vi "Test Server.vi"() -> ()   [LabVIEW 2013]
uses:
  FPGA/Rate.ctl
  <vilib>/rvi/interface/common/niFpgaWaitOnOcc.vi
  <vilib>/FPGAPlugInAG/sbRIO-9606/niLvFpga_Open_sbRIO-9606.vi
  <vilib>/rvi/interface/common/dynamic/niFpgaDynamicAddResources.vi
  <vilib>/Utility/error.llb/Error Cluster From Error Code.vi
  <vilib>/rvi/errors/niLvFpgaAdjustHostInterfaceError.vi
  <vilib>/FPGAPlugInAG/Dynamic/niLvFpga_Close_Dynamic.vi
  <vilib>/rvi/interface/nirviOpenFPGA/nirviOpenFPGA.xnode
  FPGA Bitfiles/Timothy.lvbitx
  <vilib>/rvi/interface/nirviMethod/nirviMethod.xnode
  <vilib>/rvi/interface/nirviReadWriteControl/nirviReadWriteControl.xnode
  <vilib>/rvi/interface/nirviCloseFPGA/nirviCloseFPGA.xnode
  <vilib>/rvi/errors/niLvFpgaMergeErrorWithErrorCode.vi
  <vilib>/rvi/interface/Simulation/niFpgaSimulationCallBeginRW.vi
  NiFpgaLv.dll
  <vilib>/FPGAPlugInAG/Dynamic/niLvFpga_ReadFifo_Dynamic.vi
  <vilib>/Analysis/NI_AALBase.lvlib
  Reusable/General/Math Utilities.lvlib
  <vilib>/FPGAPlugInAG/Dynamic/niLvFpga_ConfigureFifo_Dynamic.vi
  <vilib>/FPGAPlugInAG/Dynamic/niLvFpga_StartFifo_Dynamic.vi
panel:
  out "Waveform Graph 3":dbl[](graph)
  out "Delay Ticks":u32
  in  "Delay (us)":u16=16
  in  "element":dbl=16.0 format="%#_13g"
  in  "index (row)":i32
  out "Waveform Chart":cluster{i32, i32}(graph)={-1, -1}
  out "max index(es) 2":i32=-1
  out "max index(es)":i32=-1
  in  "right rank":i32=3
  out "Waveform Graph 2":i16[](graph)
  out "Exe Rate (ms)":u32=10121
  in  "Sample Time (us)":u16=100
  out "Sample Time Actual":u32
  in  "Rate":T1=8 items=["2.5 MHz"=8, "5 MHz"=4, "10 MHz"=2, "20MHz"=1]
  out "XY Graph":cluster{dbl[], dbl[]}[](graph)=[{[], []}, {[16.0, 16.0], [0.0, 0.0]}]
  out "dNewData":u64
  out "NumElements":u32
  out "samp/cycle":dbl=nan
  out "dSamps":u64
  out "Samps":u64
  in  "NumSamps":u32=100000
  out "Actual Depth":u32=1000000
  in  "Stop":bool
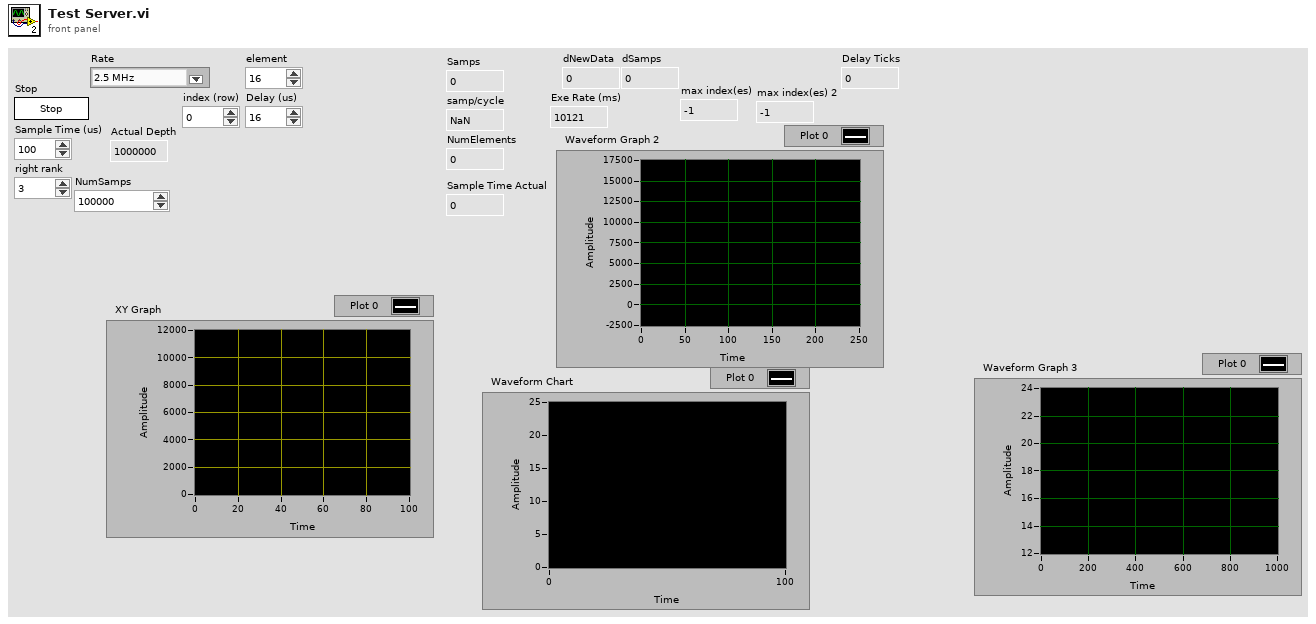
[diagram p1: front panel]
types:
  T1 = typedef "Rate.ctl" = u8
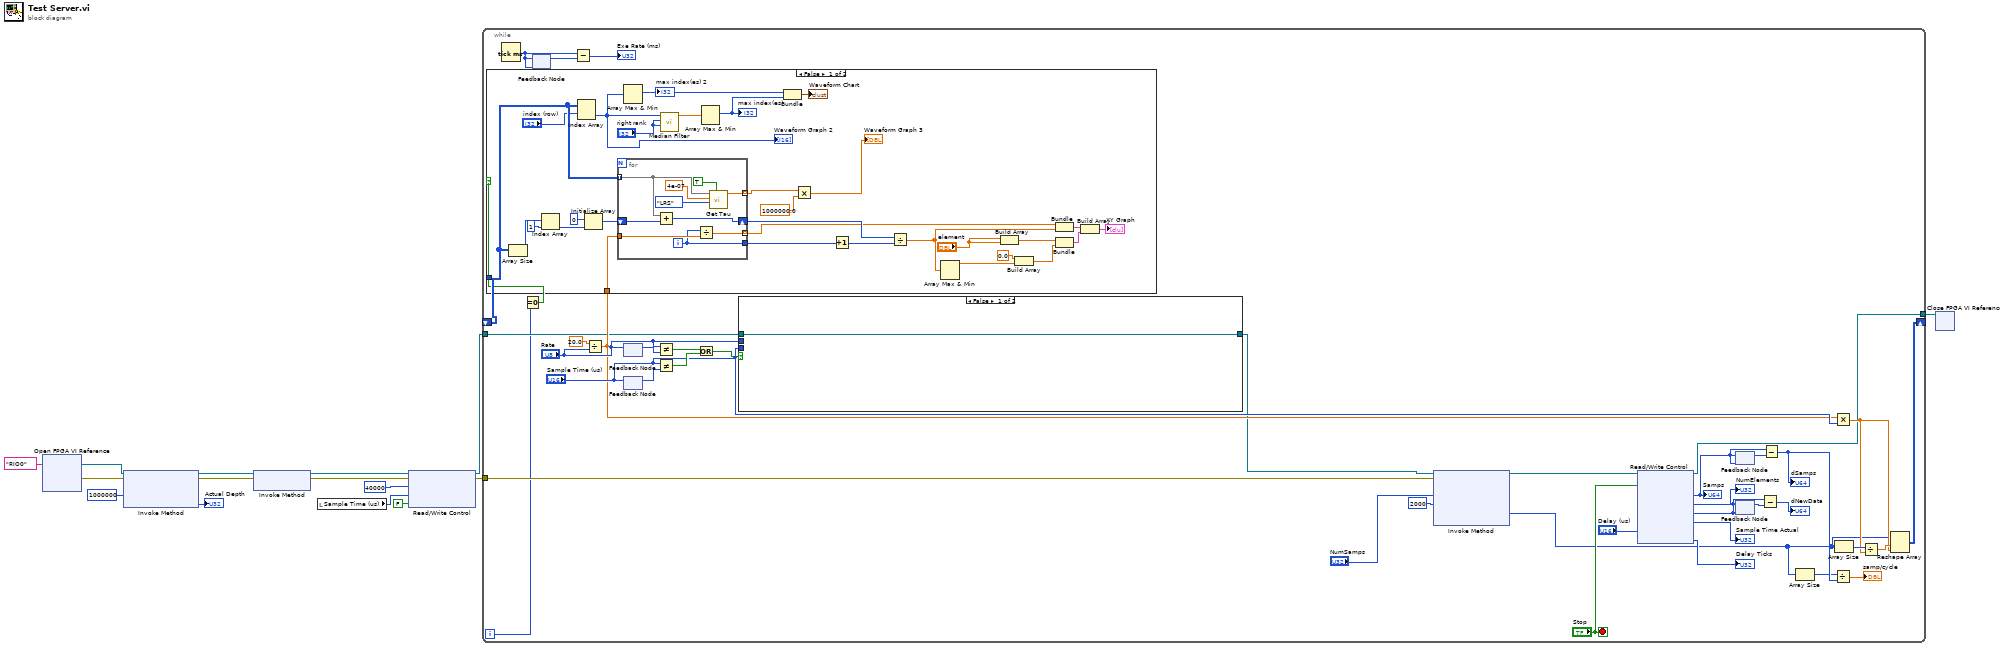
[diagram p0: block diagram]
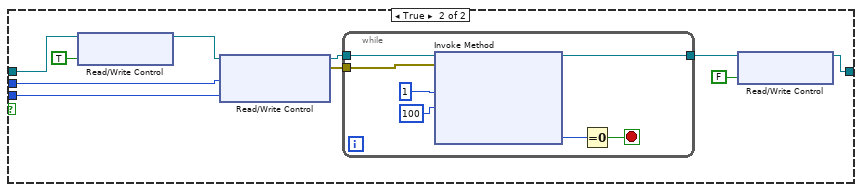
[diagram p3: hidden frame]
diagram:
  n1 = xnode "Open FPGA VI Reference"("resource name"=tag "RIO0") -> ("FPGA VI Reference Out"=w14:refnum<k20>, "error out"=w12:errorcluster)  [unwired: 1 in]
  n2 = xnode "Invoke Method"("FPGA VI Reference In"=w14, "error in"=w12, "Requested Depth"=u32 1000000) -> ("FPGA VI Reference Out"=w8:refnum<k20>, "error out"=w7:errorcluster, "Actual Depth"=→"Actual Depth":u32)
  n3 = xnode "Invoke Method"("FPGA VI Reference In"=w8, "error in"=w7) -> ("FPGA VI Reference Out"=w6:refnum<k20>, "error out"=w5:errorcluster)
  n4 = local read "Sample Time (us)"() -> (w2:u16)
  n5 = xnode "Read/Write Control"("FPGA VI Reference In"=w6, "error in"=w5, "Cylce (ticks)"=u32 40000, "Sample Time (us)"=w2, "Pause Digitizer"=FALSE) -> ("FPGA VI Reference Out"=w10:refnum<k20>, "error out"=w9:errorcluster)
  n6 = while {
    tunnel: w9 -> [w55]
    tunnel: w10 -> [w26]
    tunnel: [w24] -> w1
    shift-right: [w22] -> _
    shift-left: _ -> [w21]
    i -> [w20]
    stop <- "Stop" stop-if-true
    n7 = Tick Count (ms)() -> (millisecond timer value=w37:u32)
    n8 = Equal To 0?(x=w20) -> (x = 0?=w19:bool)
    n9 = feedback-in #1(w37) -> ()
    n10 = feedback #1(w37) -> (w36:u32)
    n11 = Subtract(x=w37, y=w36) -> (x-y=→"Exe Rate (ms)":u32)
    n12 = Divide(x=20.0, y="Rate") -> (x/y=w28:dbl)
    n13 = case shown="False" w19 {
      tunnel: w28 -> [w85 _]
      tunnel: w21 -> [w84 _]
      frame False {
        n14 = Array Size(array=w84) -> (size(s)=w77:i32[])
        n15 = Index Array(array=w77, index=1) -> (element=w75:i32)
        n16 = Index Array(array=w84, index (row)="index (row)") -> (element=w56:i16[])  [unwired: 1 in]
        "Waveform Graph 2" <- w56
        n17 = Initialize Array(0 ("index"), w75) -> (w73:i32[])
        n18 = for {
          tunnel: w84 -> [w90] mode=indexing
          shift-right: [w95] -> w72
          shift-left: w73 -> [w94]
          tunnel: [w92] -> w71
          tunnel: w85 -> [w93]
          tunnel: [w91] -> w69 mode=indexing
          tunnel: [w86] -> w59 mode=indexing
          i -> [w92]
          n19 = Add(x=w90, y=w94) -> (x+y=w95:i32[])
          n20 = Divide(x=w92, y=w93) -> (x/y=w91:dbl)
          n21 = call "Get Tau.vi"("init"=TRUE, "CalType"=enum8{"DFT-1", "DFT-5", "LRS"}."LRS", "Dt"=4e-07, "X"=w90) -> ("tau"=w86:dbl)  [unwired: 4 in, 3 out]
        }
        n22 = Array Max & Min(array=w56) -> (max index (indices)=w79:i32)  [unwired: 3 out]
        "max index(es) 2" <- w79
        n23 = call <vilib>:"Median Filter.vi"("right rank"="right rank", "left rank"="right rank", "X"=w56) -> ("Filtered X"=w81:dbl[])  [unwired: 7 in, 1 out]
        n24 = Array Max & Min(array=w81) -> (max index (indices)=w80:i32)  [unwired: 3 out]
        "max index(es)" <- w80
        n25 = Bundle(w79, w80) -> (→"Waveform Chart":cluster{i32, i32})  [unwired: 1 in]
        n26 = Multiply(x=w59, y=1000000.0 ("Dt")) -> (x*y=→"Waveform Graph 3":dbl[])
        n27 = Increment(x=w71) -> (x+1=w70:i32)
        n28 = Divide(x=w72, y=w70) -> (x/y=w68:dbl[])
        n29 = Array Max & Min(array=w68) -> (max value=w67:dbl)  [unwired: 3 out]
        n30 = Build Array("element", "element") -> (w63:dbl[])
        n31 = Build Array(0.0 ("element"), w67) -> (w66:dbl[])
        n32 = Bundle(w69, w68) -> (w62:cluster{dbl[], dbl[]})  [unwired: 1 in]
        n33 = Bundle(w63, w66) -> (w61:cluster{dbl[], dbl[]})  [unwired: 1 in]
        n34 = Build Array(w62, w61) -> (→"XY Graph":cluster{dbl[], dbl[]}[])
      }
      frame True {
      }
    }
    n35 = feedback-in #2("Rate") -> ()
    n36 = feedback #2() -> (w42:T1)  [unwired: 1 in]
    n37 = feedback #3() -> (w41:u16)  [unwired: 1 in]
    n38 = feedback-in #3("Sample Time (us)") -> ()
    n39 = Not Equal?(x="Rate", y=w42) -> (x != y?=w39:bool)
    n40 = Not Equal?(x="Sample Time (us)", y=w41) -> (x != y?=w40:bool)
    n41 = Or(x=w39, y=w40) -> (x .or. y?=w38:bool)
    n42 = case shown="False" w38 {
      tunnel: "Rate" -> [_ w106]
      tunnel: "Sample Time (us)" -> [_ w105]
      tunnel: [w96 w97] -> w25
      tunnel: w26 -> [w96 w104]
      frame False {
      }
      frame True {
        n43 = xnode "Read/Write Control"("FPGA VI Reference In"=w104, "Pause Digitizer"=TRUE) -> ("FPGA VI Reference Out"=w103:refnum<k20>)  [unwired: 1 in, 1 out]
        n44 = xnode "Read/Write Control"("FPGA VI Reference In"=w103, "Rate"=w106, "Sample Time (us)"=w105) -> ("FPGA VI Reference Out"=w101:refnum<k20>, "error out"=w100:errorcluster)  [unwired: 1 in]
        n45 = while {
          tunnel: w101 -> [w109]
          tunnel: w100 -> [w108]
          tunnel: [w107] -> w99
          stop <- w110 stop-if-true
          n46 = xnode "Invoke Method"("FPGA VI Reference In"=w109, "error in"=w108, "Number of Elements"=u32 1, "Timeout (ms)"=100) -> ("FPGA VI Reference Out"=w107:refnum<k20>, "Elements Remaining"=w111:u32)  [unwired: 2 out]
          n47 = Equal To 0?(x=w111) -> (x = 0?=w110:bool)
        }
        n48 = xnode "Read/Write Control"("FPGA VI Reference In"=w99, "Pause Digitizer"=FALSE) -> ("FPGA VI Reference Out"=w97:refnum<k20>)  [unwired: 1 in, 1 out]
      }
    }
    n49 = xnode "Invoke Method"("FPGA VI Reference In"=w25, "error in"=w55, "Number of Elements"="NumSamps", "Timeout (ms)"=2000) -> ("FPGA VI Reference Out"=w54:refnum<k20>, "Data"=w16:i16[])  [unwired: 2 out]
    n50 = xnode "Read/Write Control"("FPGA VI Reference In"=w54, "Stop"="Stop", "Delay (us)"="Delay (us)") -> ("FPGA VI Reference Out"=w24:refnum<k20>, "Samps"=w52:u64, "NumElements"=→"NumElements":u32, "NewData"=w46:u16, "Sample Ticks"=→"Sample Time Actual":u32, "Delay Ticks"=→"Delay Ticks":u32)  [unwired: 1 in, 1 out]
    "Samps" <- w52
    n51 = feedback-in #4(w52) -> ()
    n52 = feedback #4(w52) -> (w51:u64)
    n53 = feedback #5(w46) -> (w45:u16)
    n54 = feedback-in #5(w46) -> ()
    n55 = Subtract(x=w46, y=w45) -> (x-y=→"dNewData":u16)
    n56 = Subtract(x=w52, y=w51) -> (x-y=w50:u64)
    "dSamps" <- w50
    n57 = Array Size(array=w16) -> (size(s)=w47:i32)
    n58 = Divide(x=w47, y=w50) -> (x/y=→"samp/cycle":dbl)
    n59 = Multiply(x=w28, y="Sample Time (us)") -> (x*y=w31:dbl)
    n60 = Array Size(array=w16) -> (size(s)=w34:i32)
    n61 = Divide(x=w34, y=w31) -> (x/y=w32:dbl)
    n62 = Reshape Array(w16, w32, w31) -> (w22:i16[][])
  }
  n63 = xnode "Close FPGA VI Reference"("FPGA VI Reference In"=w1) -> ()  [unwired: 1 in, 1 out]
